vi "Fixing Broken Run Arrows.vi"() -> ()   [LabVIEW 2015]
panel:
  out "x2":dbl=-5.0
  out "x1":dbl=3.0
  in  "c":dbl=-15.0
  in  "b":dbl=2.0
  in  "a":dbl=1.0
  out "Area":dbl=47882219803.87908
  in  "Radius of Circle":dbl=123456.0
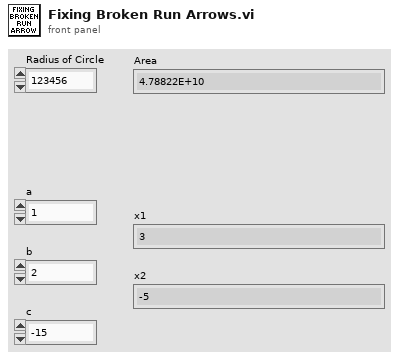
[diagram p1: front panel]
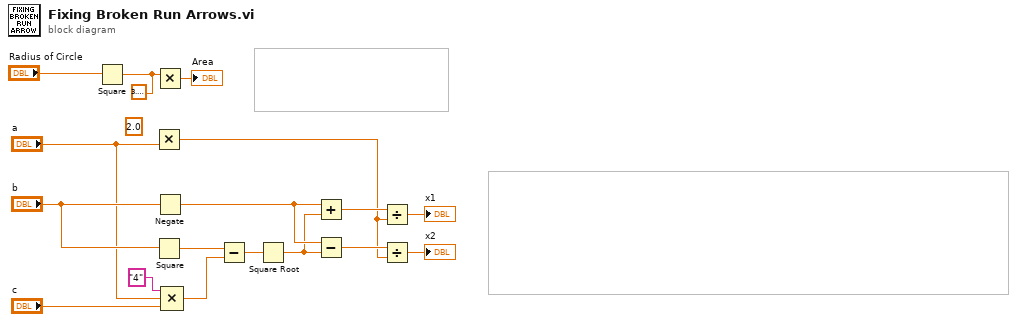
[diagram p0: block diagram]
diagram:
  (unwired) 2.0 ("x")
  w2 = 3.141592653589793
  n1 = Square(x="Radius of Circle") -> (x^2=w2:dbl)
  n2 = Multiply(y="a") -> (x*y=w4:dbl)  [unwired: 1 in]
  n3 = Square(x="b") -> (x^2=w12:dbl)
  n4 = Multiply(x=w2) -> (x*y=→"Area":dbl)  [unwired: 1 in]
  n5 = Negate(x="b") -> (-x=w7:dbl)
  n6 = Compound Arithmetic op=MULTIPLY("4", "a", "c") -> (w11:dbl)
  n7 = Subtract(x=w12, y=w11) -> (x-y=w10:dbl)
  n8 = Square Root(x=w10) -> (sqrt(x)=w6:dbl)
  n9 = Add(x=w7, y=w6) -> (x+y=w9:dbl)
  n10 = Subtract(x=w7, y=w6) -> (x-y=w5:dbl)
  n11 = Divide(x=w9, y=w4) -> (x/y=→"x1":dbl)
  n12 = Divide(x=w5, y=w4) -> (x/y=→"x2":dbl)
